vi "Error Handler ClassRef FG.vi"(7 "action (Get)":T1=enum."Get", 10 "error in (no error)":errorcluster, 11 "ErrorHandler in":refnum<class "ErrorHandler.lvclass">) -> (2 "error out":errorcluster, 3 "ErrorHandler out":refnum<class "ErrorHandler.lvclass">)   [LabVIEW 2019, in "ErrorHandler.lvclass"]
doc: "Developed by Kevin Thompson\nkevin@thompsonengineering.net\n\nCopyright 2018\nThompson Engineering, LLC"
uses:
  ErrorHandler.lvclass
  TypeDef/TD GetSet ActionSelect--enum.ctl
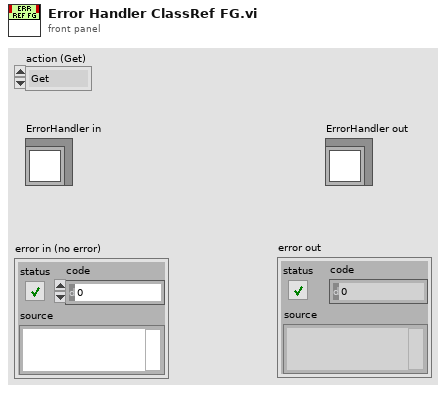
[diagram p1: front panel]
types:
  T1 = typedef "ErrorHandler.lvclass/TD GetSet ActionSelect--enum.ctl" = enum16{"Init", "Get", "Set"}
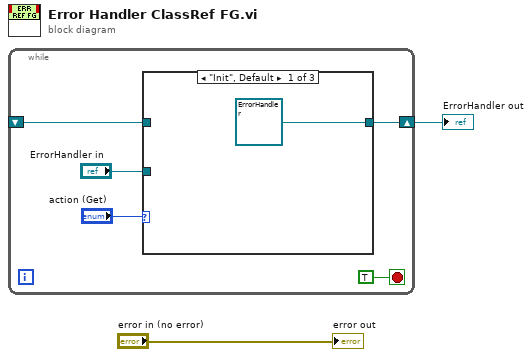
[diagram p0: block diagram]
diagram:
  n1 = while {
    shift-right: [w5] -> w2
    shift-left: _ -> [w4]
    stop <- TRUE stop-if-true
    n2 = case shown="\"Init\", Default" "action (Get)" {
      tunnel: [refnum<class "ErrorHandler.lvclass"> refnum ("ErrorHandler in") w9 w10] -> w5
      tunnel: w4 -> [_ w9 _]
      tunnel: "ErrorHandler in" -> [_ _ w10]
      frame "Init", Default {
      }
      frame "Get" {
      }
      frame "Set" {
      }
    }
  }
  "ErrorHandler out" <- w2
  "error out" <- "error in (no error)"
